vi "SetPID.vi"(4 "Gamma (-1=Use Orignal Value)":dbl=-1.0, 6 "Beta (-1=Use Orignal Value)":dbl=-1.0, 7 "Linearity (-1=Use Orignal Value)":dbl=-1.0, 8 "error in (no error)":errorcluster, 10 "PID gain schedule":T1(array[cluster]), 11 "MotorCtrl in":refnum<class "MotorControl.lvclass">) -> (0 "error out":errorcluster, 3 "MotorCtrl out":refnum<class "MotorControl.lvclass">)   [LabVIEW 2015, in "MotorControl.lvclass"]
uses:
  MotorControl.lvclass
  MotorControl.lvclass/MotorControl.ctl
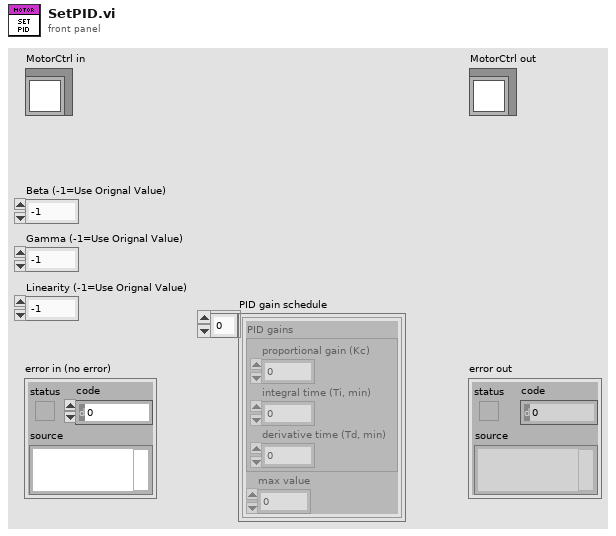
[diagram p1: front panel]
types:
  T1 = cluster{"PID gains":cluster{"proportional gain (Kc)":dbl, "integral time (Ti, min)":dbl, "derivative time (Td, min)":dbl}, "max value":dbl}[]
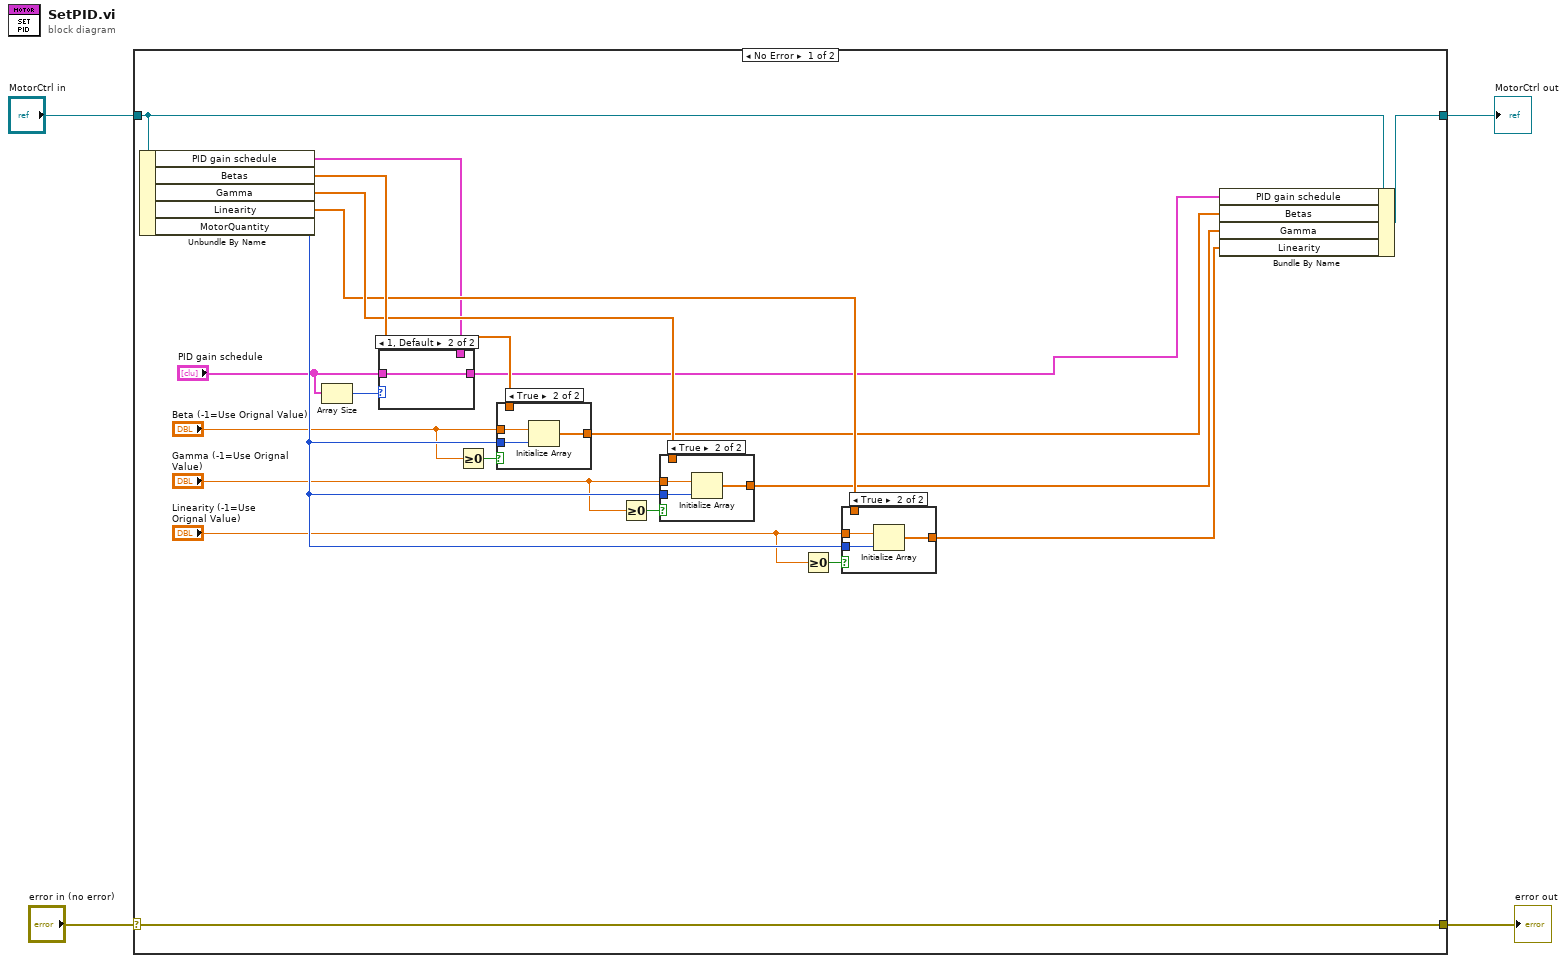
[diagram p0: block diagram]
diagram:
  n1 = case shown="No Error" "error in (no error)" {
    selector: "error in (no error)" -> [w24 w40]
    tunnel: [w24 w40] -> w3
    tunnel: [w23 w39] -> w1
    tunnel: "MotorCtrl in" -> [w22 w39]
    frame No Error {
      n2 = Unbundle By Name(w22) -> ("PID gain schedule"=w5:T1, "Betas"=w17:dbl[], "Gamma"=w16:dbl[], "Linearity"=w15:dbl[], "MotorQuantity"=w21:i32)
      n3 = Array Size(array="PID gain schedule") -> (size(s)=w8:i32)
      n4 = case shown="1, Default" w8 {
        tunnel: "PID gain schedule" -> [_ w26]
        tunnel: [w25 w26] -> w6
        tunnel: w5 -> [w25 _]
        frame 0 {
        }
        frame 1, Default {
        }
      }
      n5 = Greater Or Equal To 0?(x="Beta (-1=Use Orignal Value)") -> (x >= 0?=w11:bool)
      n6 = case shown="True" w11 {
        tunnel: "Beta (-1=Use Orignal Value)" -> [_ w38]
        tunnel: [w35 w37] -> w14
        tunnel: w21 -> [_ w36]
        tunnel: w17 -> [w35 _]
        frame False {
        }
        frame True {
          n7 = Initialize Array(w38, w36) -> (w37:dbl[])
        }
      }
      n8 = Greater Or Equal To 0?(x="Gamma (-1=Use Orignal Value)") -> (x >= 0?=w10:bool)
      n9 = case shown="True" w10 {
        tunnel: "Gamma (-1=Use Orignal Value)" -> [_ w34]
        tunnel: [w31 w33] -> w13
        tunnel: w21 -> [_ w32]
        tunnel: w16 -> [w31 _]
        frame False {
        }
        frame True {
          n10 = Initialize Array(w34, w32) -> (w33:dbl[])
        }
      }
      n11 = Greater Or Equal To 0?(x="Linearity (-1=Use Orignal Value)") -> (x >= 0?=w9:bool)
      n12 = case shown="True" w9 {
        tunnel: "Linearity (-1=Use Orignal Value)" -> [_ w30]
        tunnel: [w27 w29] -> w12
        tunnel: w21 -> [_ w28]
        tunnel: w15 -> [w27 _]
        frame False {
        }
        frame True {
          n13 = Initialize Array(w30, w28) -> (w29:dbl[])
        }
      }
      n14 = Bundle By Name(cluster=w22, "PID gain schedule"=w6, "Betas"=w14, "Gamma"=w13, "Linearity"=w12) -> (w23:refnum<class "MotorControl.lvclass">)
    }
    frame Error {
    }
  }
  "error out" <- w3
  "MotorCtrl out" <- w1
